vi "Obtain Queue.vi"(8 "error out":errorcluster) -> (0 "errorout":errorcluster, 3 "All Queue":T1)   [LabVIEW 2022 SP3]
uses:
  Controls/All Queue Ref.ctl
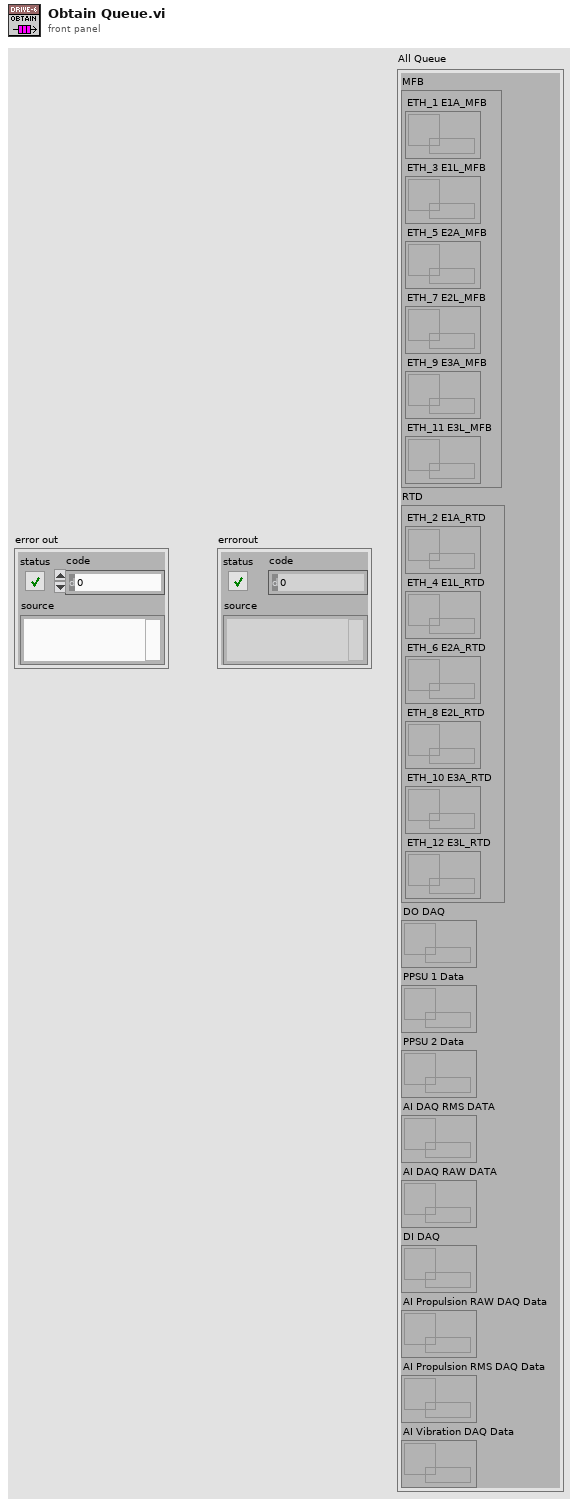
[diagram p1: front panel]
types:
  T1 = typedef "All Queue Ref.ctl" = cluster{"MFB":cluster{"ETH_1 E1A_MFB":refnum<queue>, "ETH_3 E1L_MFB":refnum<queue>, "ETH_5 E2A_MFB":refnum<queue>, "ETH_7 E2L_MFB":refnum<queue>, "ETH_9 E3A_MFB":refnum<queue>, "ETH_11 E3L_MFB":refnum<queue>}, "RTD":cluster{"ETH_2 E1A_RTD ":refnum<queue>, "ETH_4 E1L_RTD ":refnum<queue>, "ETH_6 E2A_RTD ":refnum<queue>, "ETH_8 E2L_RTD ":refnum<queue>, "ETH_10 E3A_RTD ":refnum<queue>, "ETH_12 E3L_RTD ":refnum<queue>}, "DO DAQ":refnum<queue>, "PPSU 1 Data":refnum<queue>, "PPSU 2 Data":refnum<queue>, "AI DAQ RMS DATA":refnum<queue>, "AI DAQ RAW DATA":refnum<queue>, "DI DAQ":refnum<queue>, "AI Propulsion RAW DAQ Data":refnum<queue>, "AI Propulsion RMS DAQ Data":refnum<queue>, "AI Vibration DAQ Data":refnum<queue>}
  T2 = cluster{"ETH_2 E1A_RTD ":refnum<queue>, "ETH_4 E1L_RTD ":refnum<queue>, "ETH_6 E2A_RTD ":refnum<queue>, "ETH_8 E2L_RTD ":refnum<queue>, "ETH_10 E3A_RTD ":refnum<queue>, "ETH_11 E3L_RTD ":refnum<queue>}
  T3 = cluster{"ETH_1 E1A_MFB":refnum<queue>, "ETH_3 E1L_MFB":refnum<queue>, "ETH_5 E2A_MFB":refnum<queue>, "ETH_7 E2L_MFB":refnum<queue>, "ETH_9 E3A_MFB":refnum<queue>, "ETH_11 E3L_MFB":refnum<queue>}
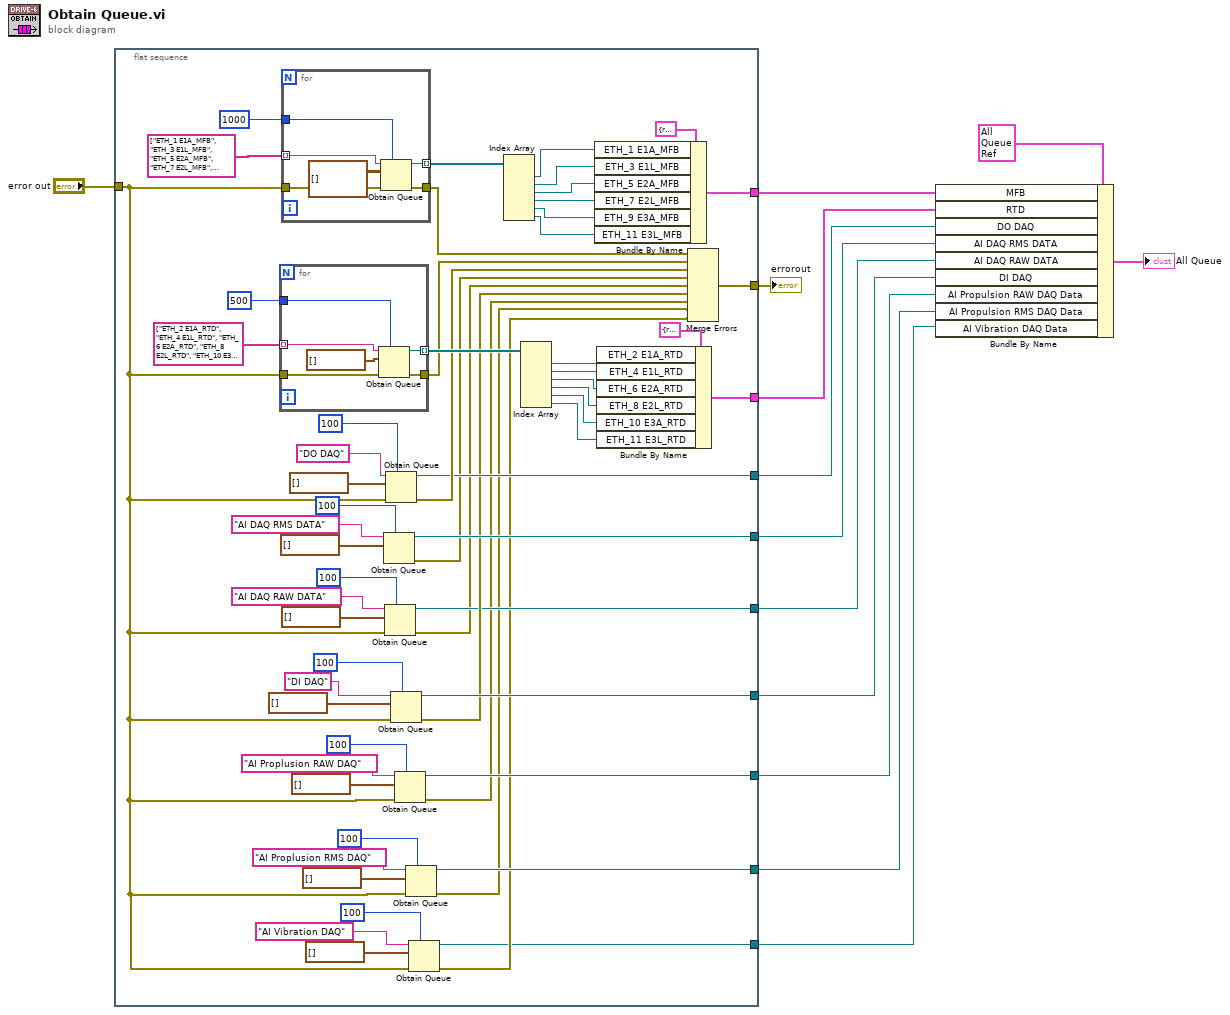
[diagram p0: block diagram]
diagram:
  n1 = flat-sequence {
    tunnel: [w54] -> w12
    tunnel: [w53] -> w11
    tunnel: "error out" -> [w17]
    tunnel: [w51] -> w8
    tunnel: [w46] -> w7
    tunnel: [w38] -> w6
    tunnel: [w37] -> w5
    tunnel: [w31] -> w4
    tunnel: [w26] -> w3
    tunnel: [w21] -> w2
    tunnel: [w14] -> w1
    frame #0 {
      n2 = for {
        tunnel: [w80] -> w50
        tunnel: [w79] -> w62 mode=indexing
        tunnel: string[] ["ETH_2 E1A_RTD", "ETH_4 E1L_RTD", "ETH_6 E2A_RTD", "ETH_8 E2L_RTD", "ETH_10 E3A_RTD", "ETH_12 E3L_RTD"] ("name (unnamed)") -> [w77] mode=indexing
        tunnel: 500 ("max queue size (-1, unlimited)") -> [w76]
        tunnel: w17 -> [w75]
        n3 = Obtain Queue(max queue size (-1, unlimited)=w76, name (unnamed)=w77, element data type=waveform(dbl)[] [] ("WF out"), error in (no error)=w75) -> (queue out=w79:refnum<queue>, error out=w80:errorcluster)  [unwired: 1 in, 1 out]
      }
      n4 = for {
        tunnel: [w86] -> w52
        tunnel: [w85] -> w71 mode=indexing
        tunnel: string[] ["ETH_1 E1A_MFB", "ETH_3 E1L_MFB", "ETH_5 E2A_MFB", "ETH_7 E2L_MFB", "ETH_9 E3A_MFB", "ETH_11 E3L_MFB"] ("name (unnamed)") -> [w83] mode=indexing
        tunnel: 1000 ("max queue size (-1, unlimited)") -> [w82]
        tunnel: w17 -> [w81]
        n5 = Obtain Queue(max queue size (-1, unlimited)=w82, name (unnamed)=w83, element data type=waveform(dbl)[][] [] ("WF out"), error in (no error)=w81) -> (queue out=w85:refnum<queue>, error out=w86:errorcluster)  [unwired: 1 in, 1 out]
      }
      n6 = Obtain Queue(max queue size (-1, unlimited)=100, name (unnamed)="AI DAQ RMS DATA", element data type=waveform(dbl)[] [] ("WF out")) -> (queue out=w38:refnum<queue>, error out=w36:errorcluster)  [unwired: 2 in, 1 out]
      n7 = Obtain Queue(max queue size (-1, unlimited)=100, name (unnamed)="AI DAQ RAW DATA", element data type=waveform(dbl)[] [] ("WF out"), error in (no error)=w17) -> (queue out=w31:refnum<queue>, error out=w30:errorcluster)  [unwired: 1 in, 1 out]
      n8 = Obtain Queue(max queue size (-1, unlimited)=100, name (unnamed)="DO DAQ", element data type=waveform(dbl)[] [] ("WF out"), error in (no error)=w17) -> (queue out=w46:refnum<queue>, error out=w47:errorcluster)  [unwired: 1 in, 1 out]
      n9 = Obtain Queue(max queue size (-1, unlimited)=100, name (unnamed)="DI DAQ", element data type=digitalwaveform[] [] ("data"), error in (no error)=w17) -> (queue out=w37:refnum<queue>, error out=w35:errorcluster)  [unwired: 1 in, 1 out]
      n10 = Obtain Queue(max queue size (-1, unlimited)=100, name (unnamed)="AI Proplusion RAW DAQ", element data type=waveform(dbl)[] [] ("WF out"), error in (no error)=w17) -> (queue out=w26:refnum<queue>, error out=w25:errorcluster)  [unwired: 1 in, 1 out]
      n11 = Obtain Queue(max queue size (-1, unlimited)=100, name (unnamed)="AI Proplusion RMS DAQ", element data type=waveform(dbl)[] [] ("WF out"), error in (no error)=w17) -> (queue out=w21:refnum<queue>, error out=w16:errorcluster)  [unwired: 1 in, 1 out]
      n12 = Obtain Queue(max queue size (-1, unlimited)=100, name (unnamed)="AI Vibration DAQ", element data type=waveform(dbl)[] [] ("WF out"), error in (no error)=w17) -> (queue out=w14:refnum<queue>, error out=w15:errorcluster)  [unwired: 1 in, 1 out]
      n13 = Index Array(array=w71) -> (element #1=w70:refnum<queue>, element #2=w69:refnum<queue>, element #3=w68:refnum<queue>, element #4=w67:refnum<queue>, element #5=w66:refnum<queue>, element #6=w65:refnum<queue>)  [unwired: 6 in]
      n14 = Index Array(array=w62) -> (element #1=w60:refnum<queue>, element #2=w59:refnum<queue>, element #3=w58:refnum<queue>, element #4=w57:refnum<queue>, element #5=w56:refnum<queue>, element #6=w55:refnum<queue>)  [unwired: 6 in]
      n15 = Bundle By Name(cluster=T3 {"ETH_1 E1A_MFB"=refnum, "ETH_3 E1L_MFB"=refnum, "ETH_5 E2A_MFB"=refnum, "ETH_7 E2L_MFB"=refnum, "ETH_9 E3A_MFB"=refnum, "ETH_11 E3L_MFB"=refnum}, "ETH_1 E1A_MFB"=w70, "ETH_3 E1L_MFB"=w69, "ETH_5 E2A_MFB"=w68, "ETH_7 E2L_MFB"=w67, "ETH_9 E3A_MFB"=w66, "ETH_11 E3L_MFB"=w65) -> (w54:T3)
      n16 = Bundle By Name(cluster=T2 {"ETH_2 E1A_RTD "=refnum, "ETH_4 E1L_RTD "=refnum, "ETH_6 E2A_RTD "=refnum, "ETH_8 E2L_RTD "=refnum, "ETH_10 E3A_RTD "=refnum, "ETH_11 E3L_RTD "=refnum}, "ETH_2 E1A_RTD"=w60, "ETH_4 E1L_RTD"=w59, "ETH_6 E2A_RTD"=w58, "ETH_8 E2L_RTD"=w57, "ETH_10 E3A_RTD"=w56, "ETH_11 E3L_RTD"=w55) -> (w53:T2)
      n17 = Merge Errors(w52, w50, w47, w36, w30, w35, w25, w16, w15) -> (w51:errorcluster)
    }
  }
  n18 = Bundle By Name(cluster=T1 {"MFB"={"ETH_1 E1A_MFB"=refnum, "ETH_3 E1L_MFB"=refnum, "ETH_5 E2A_MFB"=refnum, "ETH_7 E2L_MFB"=refnum, "ETH_9 E3A_MFB"=refnum, "ETH_11 E3L_MFB"=refnum}, "RTD"={"ETH_2 E1A_RTD "=refnum, "ETH_4 E1L_RTD "=refnum, "ETH_6 E2A_RTD "=refnum, "ETH_8 E2L_RTD "=refnum, "ETH_10 E3A_RTD "=refnum, "ETH_12 E3L_RTD "=refnum}, "DO DAQ"=refnum, "PPSU 1 Data"=refnum, "PPSU 2 Data"=refnum, "AI DAQ RMS DATA"=refnum, "AI DAQ RAW DATA"=refnum, "DI DAQ"=refnum, "AI Propulsion RAW DAQ Data"=refnum, "AI Propulsion RMS DAQ Data"=refnum, "AI Vibration DAQ Data"=refnum} ("Queue"), "MFB"=w12, "RTD"=w11, "DO DAQ"=w7, "AI DAQ RMS DATA"=w6, "AI DAQ RAW DATA"=w4, "DI DAQ"=w5, "AI Propulsion RAW DAQ Data"=w3, "AI Propulsion RMS DAQ Data"=w2, "AI Vibration DAQ Data"=w1) -> (→"All Queue":T1)
  "errorout" <- w8
